vi "SlaveState.vi"(0 "Strings in":string[](array[string])=["C:\\CuspControl\\GPIB and Network\\Cusp\\SlaveState.txt"], 1 "Dubs in":dbl[](array[numeric])=[0.0]) -> ()   [LabVIEW 2018]
panel:
  in  "subvi":bool=TRUE
  in  "Slave state":dbl
  in  "Inbit file":path=path "C:/CuspControl/GPIB and Network/Cusp/SlaveState.txt"
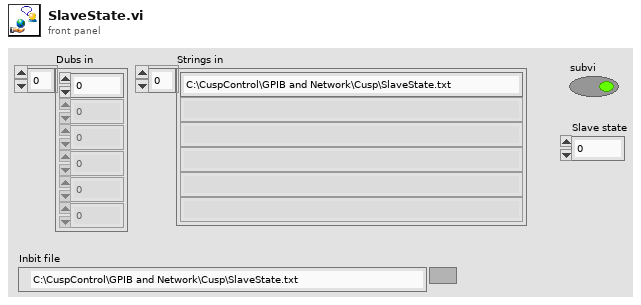
[diagram p1: front panel]
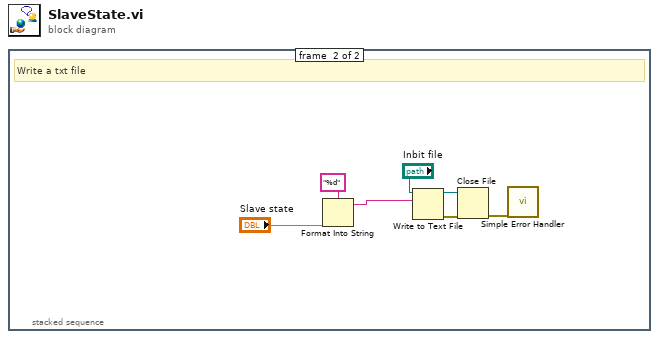
[diagram p0: block diagram]
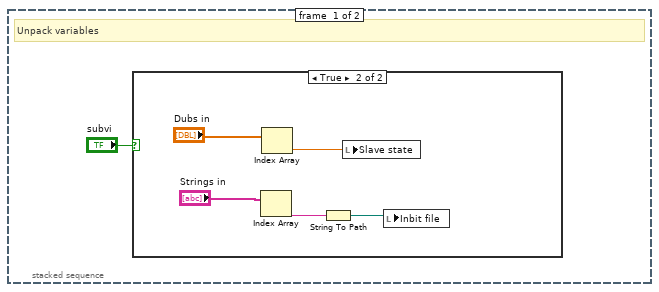
[diagram p2: hidden frame]
diagram:
  n1 = stacked-sequence {
    frame #0 {
      # "Unpack variables"
      n2 = case shown="True" "subvi" {
        frame False {
        }
        frame True {
          n3 = Index Array(array="Strings in") -> (element=w3:string)  [unwired: 1 in]
          n4 = Index Array(array="Dubs in") -> (element=w4:dbl)  [unwired: 1 in]
          n5 = String To Path(string=w3) -> (path=w2:path)
          n6 = local write "Slave state"(w4) -> ()
          n7 = local write "Inbit file"(w2) -> ()
        }
      }
    }
    frame #1 {
      # "Write a txt file"
      n8 = Format Into String(format string="%d", "Slave state") -> (resulting string=w7:string)  [unwired: 2 in, 1 out]
      n9 = Write to Text File(file (use dialog)="Inbit file", text=w7) -> (refnum out=w9:refnum<file>, error out=w10:errorcluster)  [unwired: 2 in, 1 out]
      n10 = Close File(refnum=w9, error in=w10) -> (error out=w8:errorcluster)  [unwired: 1 out]
      n11 = call <vilib>:"Simple Error Handler.vi"("error in (no error)"=w8) -> ()  [unwired: 4 in, 5 out]
    }
  }
